vi "vsTimeWindow.vi"() -> ()   [LabVIEW 2020]
uses:
  <vilib>/Math Plots/2D Math Plots/2D Error Bar/2D Error Bar XCtrl/2D Error Bar.xctl
  C:/Program Files/Dotfast Consulting/Timetag Explorer 2.26/ttInterface.dll
  Program Files/Dotfast Consulting/Timetag Explorer 2.26/ttInterface.dll
  <vilib>/Utility/file.llb/Write Delimited Spreadsheet (I64).vi
  <vilib>/Math Plots/2D Math Plots/2D Error Bar/2D Error Bar Datatype/Public/Plot Helper (Fixed).vi
  <vilib>/gmath/statdist.llb/st_Percentiles (scalar).vi
  <vilib>/Analysis/NI_AALBase.lvlib
  <vilib>/Math Plots/2D Math Plots/2D Error Bar/2D Error Bar Datatype/2D Error Bar Datatype.lvclass
  <vilib>/gmath/NI_Gmath.lvlib
panel:
  out "Ratio":dbl format="%#_6p"
  out "Peak":dbl format="%#_6p"
  out "BackGround":dbl format="%#_6p"
  in  "stop":bool
  in  "Boolean":bool=TRUE
  in  "Step Delay(ns)":dbl
  in  "Stop Delay (ns)":dbl
  in  "StartDelay (ns)":dbl
  in  "fileName":string
  in  "Folder":path
  out "ChB Delay (uqd Unit)":i32
  out "ChADelay(uqd Unit)":i32
  in  "chB delay (ns)":dbl
  in  "chA delay(ns)":dbl
  in  "Ch B":u8=1 min=1 max=16 step=1
  in  "Ch A":u8=1 min=1 max=16 step=1
  out "CTW (uqd units)":i32
  in  "CTW in ns":dbl
  out "2D Error Bar":refnum<class "2D Plot Datatype.lvclass">[](xcontrol)
  out "Coincidence Rate AvsB":dbl format="%#_4p"
  out "ChB Rate":dbl format="%#_4p"
  out "ChARate":dbl format="%#_4p"
  out "Coincidence AvsB":i32
  out "Ch A":i32
  out "GetTimeCounter":i32
  out "Ch B":i32
  out "GetResolution":dbl
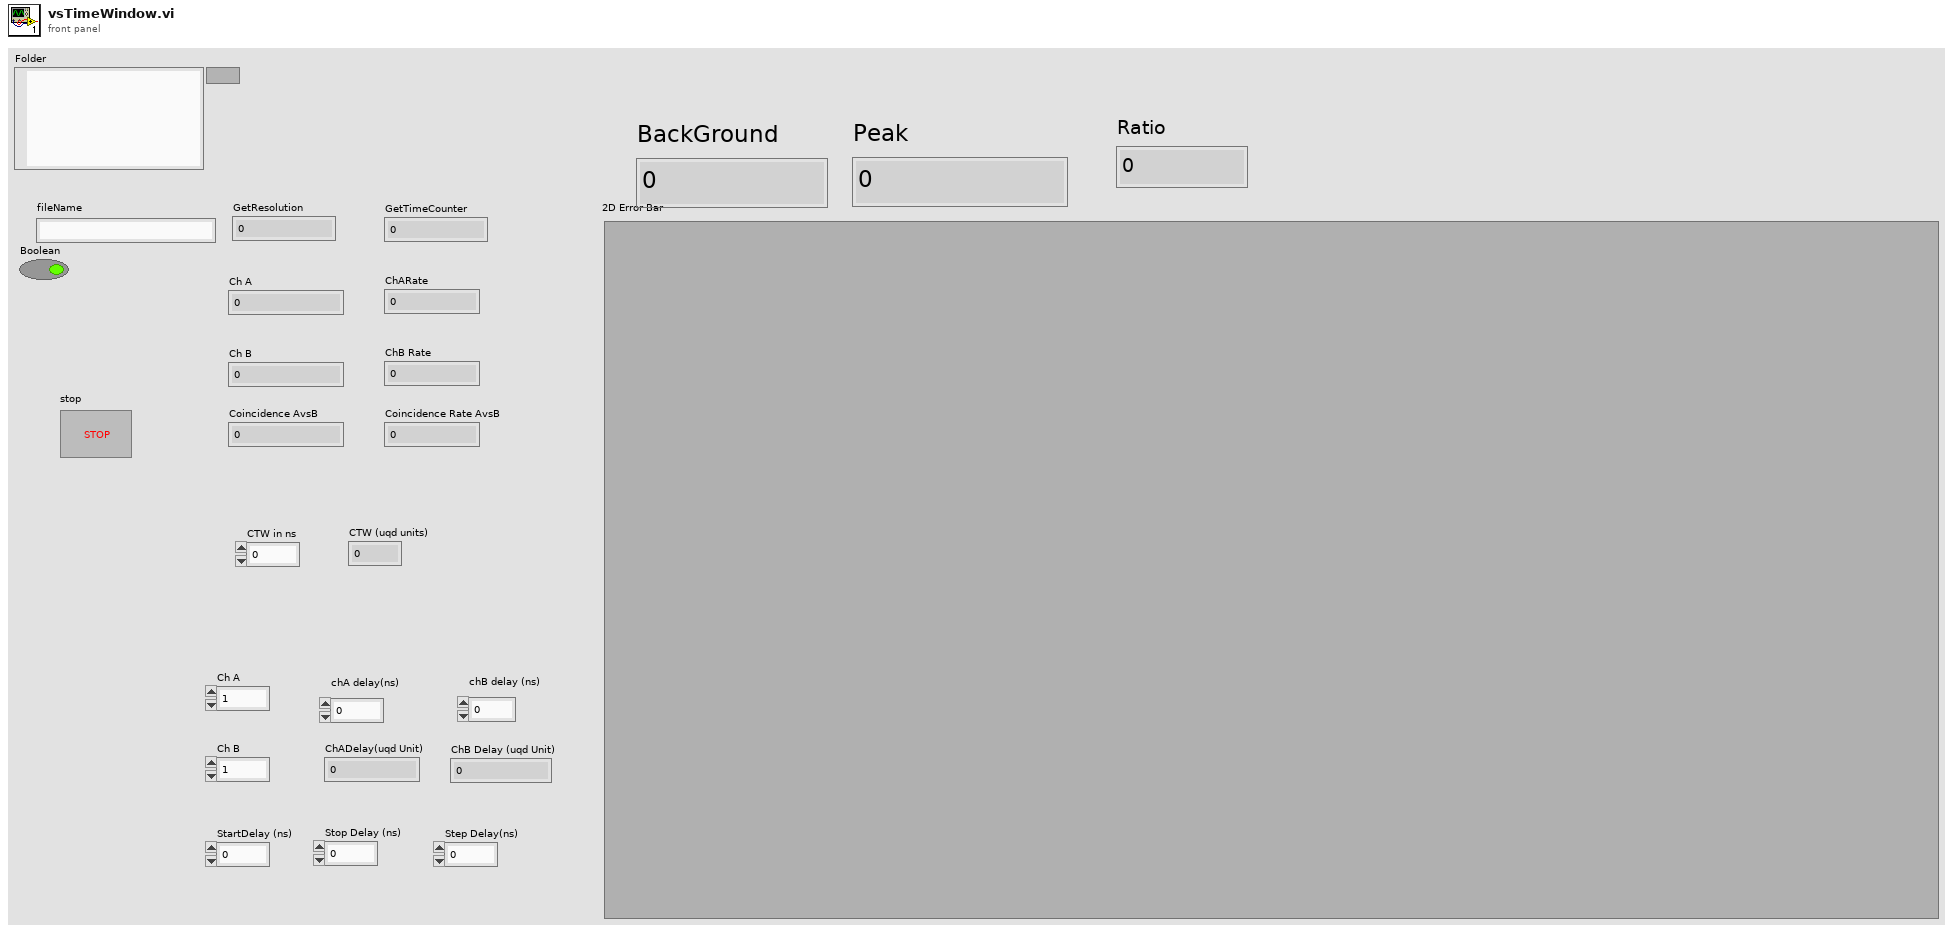
[diagram p1: front panel]
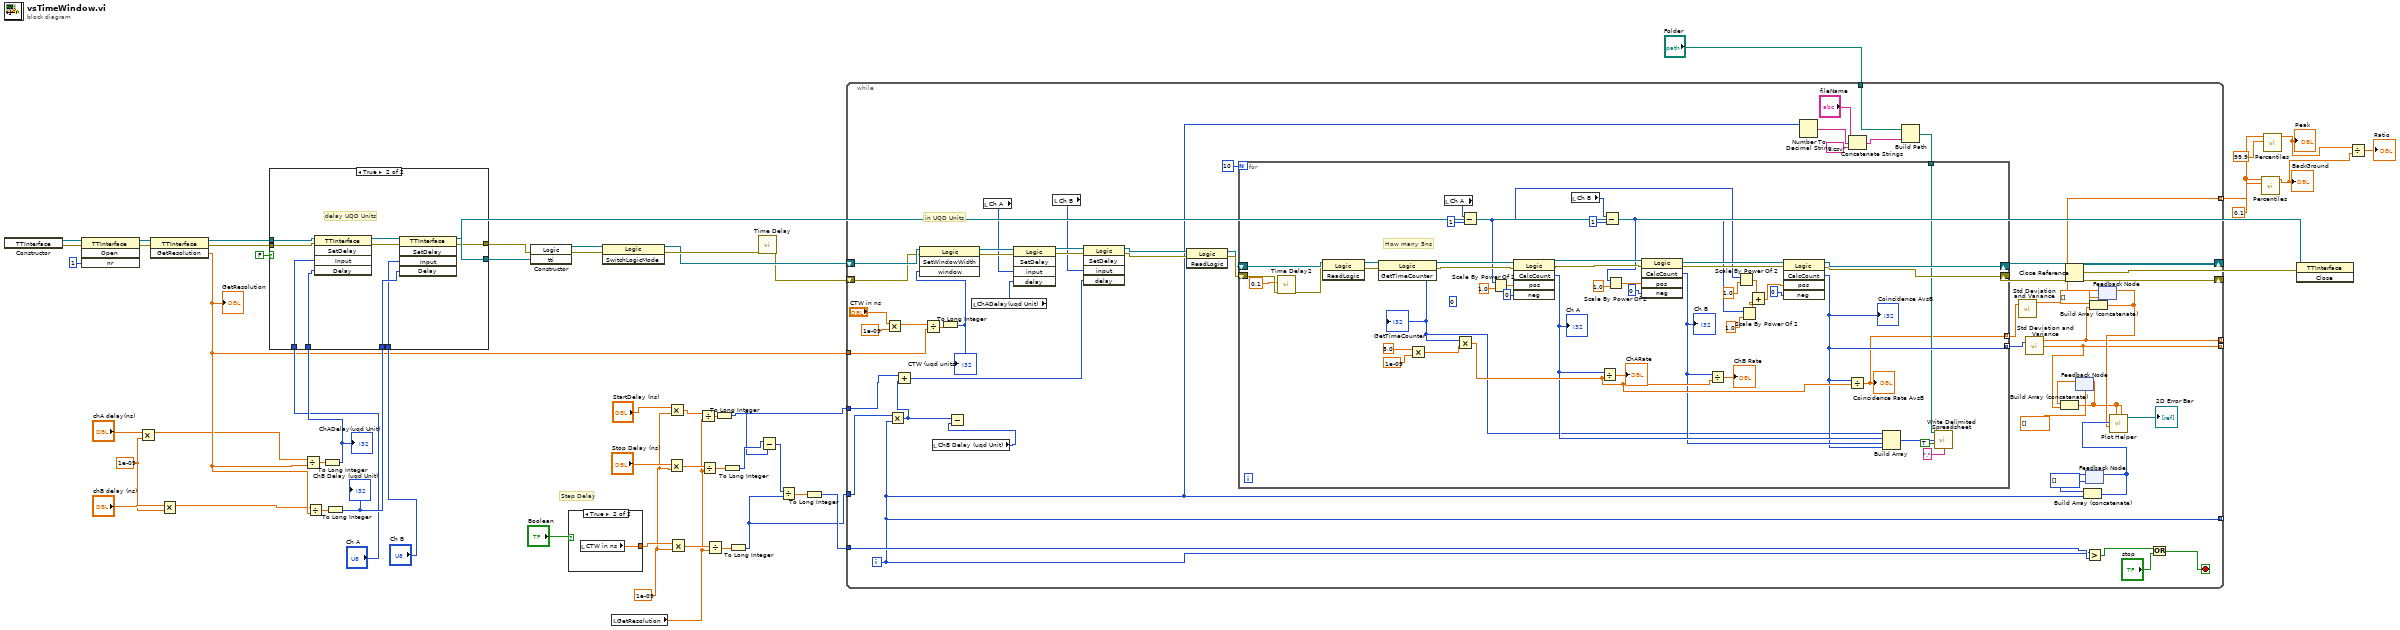
[diagram p0: block diagram]
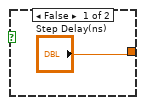
[diagram p2: hidden frame]
diagram:
  w20 = 1e-09
  w26 = 1e-09
  # "Step Delay"
  n1 = constructor class="TTInterface"() -> (reference out=w55:refnum<k24>, error out=w54:errorcluster)  [unwired: 3 in, 1 out]
  n2 = invoke class="TTInterface" method="Open"(reference=w55, error in=w54, "nr"=1) -> (reference out=w51:refnum<k24>, error out=w52:errorcluster)  [unwired: 1 in, 2 out]
  n3 = Multiply(x="chA delay(ns)", y=w26) -> (x*y=w28:dbl)
  n4 = invoke class="TTInterface" method="GetResolution"(reference=w51, error in=w52) -> (reference out=w50:refnum<k24>, error out=w49:errorcluster, "GetResolution"=w29:dbl)  [unwired: 1 in]
  "GetResolution" <- w29
  n5 = Multiply(x="chB delay (ns)", y=w26) -> (x*y=w27:dbl)
  n6 = Divide(x=w28, y=w29) -> (x/y=w35:dbl)
  n7 = Divide(x=w27, y=w29) -> (x/y=w34:dbl)
  n8 = To Long Integer(number=w35) -> (32bit integer=w33:i32)
  "ChADelay(uqd Unit)" <- w33
  n9 = To Long Integer(number=w34) -> (32bit integer=w32:i32)
  "ChB Delay (uqd Unit)" <- w32
  n10 = case shown="True" FALSE {
    tunnel: w50 -> [w57 w67]
    tunnel: w49 -> [w56 w66]
    tunnel: [w56 w63] -> w48
    tunnel: [w57 w62] -> w45
    tunnel: w33 -> [_ w61]
    tunnel: w32 -> [_ w60]
    tunnel: "Ch A" -> [_ w59]
    tunnel: "Ch B" -> [_ w58]
    frame False {
    }
    frame True {
      # "delay UQD Units"
      n11 = invoke class="TTInterface" method="SetDelay"(reference=w67, error in=w66, "Input"=w59, "Delay"=w61) -> (reference out=w65:refnum<k24>, error out=w64:errorcluster)  [unwired: 1 in, 3 out]
      n12 = invoke class="TTInterface" method="SetDelay"(reference=w65, error in=w64, "Input"=w58, "Delay"=w60) -> (reference out=w62:refnum<k24>, error out=w63:errorcluster)  [unwired: 1 in, 3 out]
    }
  }
  n13 = constructor class="Logic"(error in=w48, "tti"=w45) -> (reference out=w47:refnum<k24>, error out=w46:errorcluster)  [unwired: 2 in, 2 out]
  n14 = case shown="True" "Boolean" {
    tunnel: ["Step Delay(ns)" w69] -> w21
    frame False {
    }
    frame True {
      n15 = local read "CTW in ns"() -> (w69:dbl)
    }
  }
  n16 = invoke class="Logic" method="SwitchLogicMode"(reference=w47, error in=w46) -> (reference out=w40:refnum<k24>, error out=w41:errorcluster)  [unwired: 1 in, 1 out]
  n17 = local read "GetResolution"() -> (w16:dbl)
  n18 = Multiply(x="Stop Delay (ns)", y=w20) -> (x*y=w17:dbl)
  n19 = Multiply(x="StartDelay (ns)", y=w20) -> (x*y=w19:dbl)
  n20 = Multiply(x=w21, y=w20) -> (x*y=w18:dbl)
  n21 = Divide(x=w19, y=w16) -> (x/y=w15:dbl)
  n22 = Divide(x=w17, y=w16) -> (x/y=w14:dbl)
  n23 = Divide(x=w18, y=w16) -> (x/y=w13:dbl)
  n24 = To Long Integer(number=w15) -> (32bit integer=w9:i32)
  n25 = To Long Integer(number=w14) -> (32bit integer=w10:i32)
  n26 = To Long Integer(number=w13) -> (32bit integer=w7:i32)
  n27 = call "Time Delay"("error in (no error)"=w41) -> ("error out"=w39:errorcluster)  [unwired: 10 in]
  n28 = Subtract(x=w10, y=w9) -> (x-y=w12:i32)
  n29 = Divide(x=w12, y=w7) -> (x/y=w11:dbl)
  n30 = To Long Integer(number=w11) -> (32bit integer=w8:i32)
  n31 = while {
    shift-right: [w122] -> w43
    shift-left: w40 -> [w117]
    shift-right: [w121] -> w42
    shift-left: w39 -> [w116]
    tunnel: [w71] -> _ mode=indexing
    tunnel: [w96] -> _ mode=indexing
    tunnel: [w77] -> _ mode=indexing
    tunnel: w29 -> [w107]
    tunnel: "Folder" -> [w90]
    tunnel: w9 -> [w76]
    tunnel: w8 -> [w81]
    tunnel: w7 -> [w78]
    tunnel: [w72] -> w5 mode=indexing
    i -> [w77]
    stop <- w83 stop-if-true
    # "in UQD Units"
    n32 = Multiply(x="CTW in ns", y=1e-09) -> (x*y=w106:dbl)
    n33 = Multiply(x=w78, y=w77) -> (x*y=w75:i32)
    n34 = Add(x=w76, y=w75) -> (x+y=w74:i32)
    n35 = Divide(x=w106, y=w107) -> (x/y=w108:dbl)
    n36 = local read "ChB Delay (uqd Unit)"() -> (w84:i32)
    n37 = To Long Integer(number=w108) -> (32bit integer=w104:i32)
    "CTW (uqd units)" <- w104
    n38 = invoke class="Logic" method="SetWindowWidth"(reference=w117, error in=w116, "window"=w104) -> (reference out=w115:refnum<k24>, error out=w114:errorcluster)  [unwired: 1 in, 2 out]
    n39 = Subtract(x=w75, y=w84) -> ()  [unwired: 1 out]
    n40 = local read "ChADelay(uqd Unit)"() -> (w79:i32)
    n41 = local read "Ch A"() -> (w92:u8)
    n42 = invoke class="Logic" method="SetDelay"(reference=w115, error in=w114, "input"=w92, "delay"=w79) -> (reference out=w111:refnum<k24>, error out=w110:errorcluster)  [unwired: 1 in, 3 out]
    n43 = local read "Ch B"() -> (w91:u8)
    n44 = invoke class="Logic" method="SetDelay"(reference=w111, error in=w110, "input"=w91, "delay"=w74) -> (reference out=w113:refnum<k24>, error out=w112:errorcluster)  [unwired: 1 in, 3 out]
    n45 = invoke class="Logic" method="ReadLogic"(reference=w113, error in=w112) -> (reference out=w119:refnum<k24>, error out=w120:errorcluster)  [unwired: 1 in, 1 out]
    n46 = Number To Decimal String(number=w77) -> (decimal integer string=w87:string)  [unwired: 1 in]
    n47 = Concatenate Strings("fileName", w87, ".csv" ("string")) -> (w88:string)
    n48 = Build Path(base path=w90, name or relative path=w88) -> (appended path=w89:path)
    n49 = for {
      N: 10 -> [_]
      shift-right: [w146] -> w121
      shift-left: w120 -> [w166]
      shift-right: [w147] -> w122
      shift-left: w119 -> [w165]
      tunnel: [w129] -> w73 mode=indexing
      tunnel: w89 -> [w124]
      tunnel: [w123] -> w70 mode=indexing
      (unwired) u8 0 ("y")
      # "How many 5ns"
      n50 = call "Time Delay2"("error in (no error)"=w166, "Delay Time (s)"=0.1) -> ("error out"=w164:errorcluster)  [unwired: 9 in]
      n51 = invoke class="Logic" method="ReadLogic"(reference=w165, error in=w164) -> (reference out=w159:refnum<k24>, error out=w158:errorcluster)  [unwired: 1 in, 1 out]
      n52 = invoke class="Logic" method="GetTimeCounter"(reference=w159, error in=w158) -> (reference out=w154:refnum<k24>, error out=w153:errorcluster, "GetTimeCounter"=w127:i32)  [unwired: 1 in]
      "GetTimeCounter" <- w127
      n53 = Multiply(x=5.0, y=1e-09) -> (x*y=w160:dbl)
      n54 = local read "Ch A"() -> (w138:u8)
      n55 = Multiply(x=w127, y=w160) -> (x*y=w132:dbl)
      n56 = Subtract(x=w138, y=u8 1) -> (x-y=w134:u8)
      n57 = Scale By Power Of 2(n=w134, x=1.0) -> (x*2^n=w156:dbl)
      n58 = invoke class="Logic" method="CalcCount"(reference=w154, error in=w153, "pos"=w156, "neg"=0) -> (reference out=w152:refnum<k24>, error out=w151:errorcluster, "CalcCount"=w131:i32)  [unwired: 1 in, 2 out]
      "Ch A" <- w131
      n59 = local read "Ch B"() -> (w136:u8)
      n60 = Divide(x=w131, y=w132) -> (x/y=→"ChARate":dbl)
      n61 = Subtract(x=w136, y=u8 1) -> (x-y=w133:u8)
      n62 = Scale By Power Of 2(n=w133, x=1.0) -> (x*2^n=w168:dbl)
      n63 = invoke class="Logic" method="CalcCount"(reference=w152, error in=w151, "pos"=w168, "neg"=0) -> (reference out=w149:refnum<k24>, error out=w148:errorcluster, "CalcCount"=w130:i32)  [unwired: 1 in, 2 out]
      "Ch B" <- w130
      n64 = Divide(x=w130, y=w132) -> (x/y=→"ChB Rate":dbl)
      n65 = Scale By Power Of 2(n=w134, x=1.0) -> (x*2^n=w143:dbl)
      n66 = Scale By Power Of 2(n=w133, x=1.0) -> (x*2^n=w142:dbl)
      n67 = Add(x=w143, y=w142) -> (x+y=w141:dbl)
      n68 = invoke class="Logic" method="CalcCount"(reference=w149, error in=w148, "pos"=w141, "neg"=0) -> (reference out=w147:refnum<k24>, error out=w146:errorcluster, "CalcCount"=w129:i32)  [unwired: 1 in, 2 out]
      "Coincidence AvsB" <- w129
      n69 = Divide(x=w129, y=w132) -> (x/y=w123:dbl)
      "Coincidence Rate AvsB" <- w123
      n70 = Build Array(w127, w131, w130, w129) -> (w128:i32[])
      n71 = call-poly <vilib>:"Write Delimited Spreadsheet.vi"("file path (dialog if empty)"=w124, "1D data"=w128, "append to file? (new file:F)"=TRUE, "delimiter (\\t)"="," ("delimiter (\\t)")) -> ()  [unwired: 10 in, 2 out]
    }
    n72 = call <vilib>:"Std Deviation and Variance.vi"("X"=w70) -> ("mean"=w72:dbl)  [unwired: 1 in, 2 out]
    n73 = call <vilib>:"Std Deviation and Variance.vi"("X"=w73) -> ("mean"=w71:dbl, "standard deviation"=w96:dbl)  [unwired: 1 in, 1 out]
    n74 = feedback #1(dbl[] []) -> (w95:dbl[])
    n75 = Build Array (concatenate)(w95, w96) -> (w93:dbl[])
    n76 = feedback-in #1(w93) -> ()
    n77 = feedback #2(i32[] []) -> (w102:i32[])
    n78 = Build Array (concatenate)(w102, w77) -> (w100:i32[])
    n79 = feedback-in #2(w100) -> ()
    n80 = Greater?(x=w77, y=w81) -> (0:w80:bool)
    n81 = feedback #3(dbl[] []) -> (w99:dbl[])
    n82 = Build Array (concatenate)(w99, w71) -> (w98:dbl[])
    n83 = feedback-in #3(w98) -> ()
    n84 = call-poly <vilib>:"Plot Helper.vi"("error b vector"=w93, "error a vector"=w93, "y vector"=w98, "x vector"=w100) -> ("2D Plot Class Obj Array out"=→"2D Error Bar":refnum<class "2D Plot Datatype.lvclass">[])  [unwired: 2 in, 5 out]
    n85 = Or(x=w80, y="stop") -> (x .or. y?=w83:bool)
  }
  n86 = Close Reference(reference=w43, error in (no error)=w42) -> (error out=w44:errorcluster)
  n87 = call-poly <vilib>:"Percentiles.vi"("p"=0.1, "x array"=w5) -> ("percentile"=w2:dbl)  [unwired: 8 in, 1 out]
  "BackGround" <- w2
  n88 = call-poly <vilib>:"Percentiles.vi"("p"=99.9, "x array"=w5) -> ("percentile"=w3:dbl)  [unwired: 8 in, 1 out]
  "Peak" <- w3
  n89 = invoke class="TTInterface" method="Close"(reference=w45, error in=w44) -> ()  [unwired: 1 in, 3 out]
  n90 = Divide(x=w3, y=w2) -> (x/y=→"Ratio":dbl)
